vi "UDP Data Link - RTMs - Remove Unbound Channels.vi"(8 "error in (no error)":errorcluster, 11 "Node Ptr":u64 format="%.0x") -> (0 "error out":errorcluster)   [LabVIEW 2016, in "UDP-Custom-Device System Explorer.lvlib"]
uses:
  UDP-Custom-Device System Explorer.lvlib
  <vilib>/NI VeriStand/Custom Device API/Custom Device API.lvlib
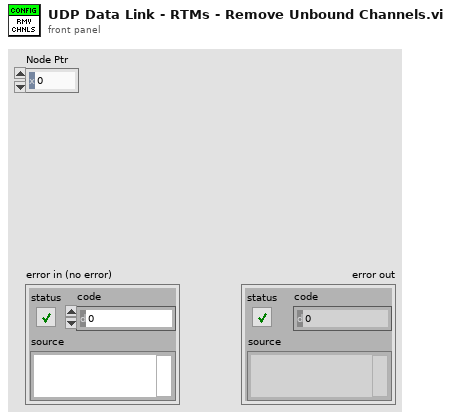
[diagram p1: front panel]
types:
  T1 = typedef "Custom Device API.lvlib/Custom Device Item Ref.ctl" = u64
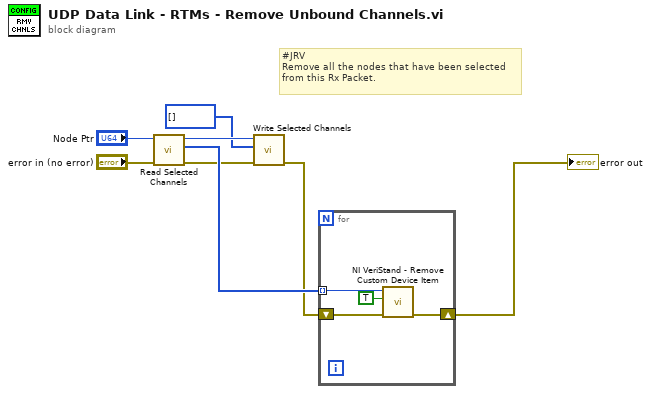
[diagram p0: block diagram]
diagram:
  # "#JRV\nRemove all the nodes that have been selected\nfrom this Rx Packet."
  n1 = call "Read Selected Channels.vi"("error in (no error)"="error in (no error)", "Node Ptr"="Node Ptr") -> ("error out"=w3:errorcluster, "Selected Channel References"=w5:u64[], "Node Ptr out"=w4:T1)  [unwired: 7 in]
  n2 = call "Write Selected Channels.vi"("error in (no error)"=w3, "Selected Channel References"=u64[] [], "Node Ptr"=w4) -> ("error out"=w2:errorcluster)  [unwired: 7 in, 1 out]
  n3 = for {
    shift-right: [w11] -> w6
    shift-left: w2 -> [w12]
    tunnel: w5 -> [w10] mode=indexing
    n4 = call <vilib>:"NI VeriStand - Remove Custom Device Item.vi"("error in (no error)"=w12, "Force Delete (F)"=TRUE, "Item Ref in"=w10) -> ("error out"=w11:errorcluster)  [unwired: 7 in, 1 out]
  }
  "error out" <- w6
